vi "Fridge_Valve_Global.vi"() -> ()   [LabVIEW 2019]
panel:
  out "FV_nose_level":dbl
  out "FV_bypass_valve":dbl
  out "FV_ST":u32(colorbox)
  out "FV_run_valve":dbl
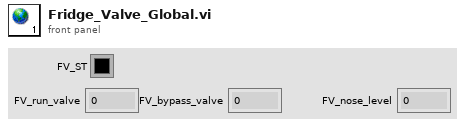
[diagram p1: front panel]
diagram:
